vi "Anti-Tip Log.vi"   [LabVIEW 2014]
uses:
  <vilib>/Rock Robotics/Network Tables/SD Read Boolean.vi
  Begin/Global Variables.vi
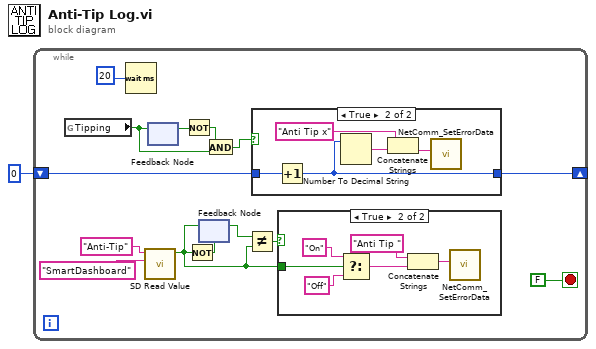
[diagram p0: block diagram]
diagram:
  n1 = while {
    shift-right: [w9] -> _
    shift-left: i16 0 ("width (-)") -> [w10]
    stop <- FALSE stop-if-true
    n2 = global read "Global Variables.vi" "Tipping"() -> (w13:bool)
    n3 = Wait (ms)(milliseconds to wait=u32 20) -> ()  [unwired: 1 out]
    n4 = call-poly <vilib>:"SD Read Value.vi"("Table Prefix"="SmartDashboard", "Name"="Anti-Tip") -> ("Boolean"=w2:bool)  [unwired: 7 in, 2 out]
    n5 = feedback-in #1(w13) -> ()
    n6 = feedback #1() -> (w15:bool)  [unwired: 1 in]
    n7 = Not(x=w15) -> (.not. x?=w14:bool)
    n8 = Not(x=w2) -> (.not. x?=w3:bool)
    n9 = feedback #2(w3) -> (w5:bool)
    n10 = feedback-in #2(w2) -> ()
    n11 = And(x=w14, y=w13) -> (x .and. y?=w12:bool)
    n12 = Not Equal?(x=w5, y=w2) -> (x != y?=w4:bool)
    n13 = case shown="True" w12 {
      tunnel: w10 -> [w22 w24]
      tunnel: [w22 w23] -> w9
      frame False {
      }
      frame True {
        n14 = Increment(x=w24) -> (x+1=w23:i16)
        n15 = Number To Decimal String(number=w23) -> (decimal integer string=w25:string)  [unwired: 1 in]
        n16 = Concatenate Strings("Anti Tip x" ("Error Data"), w25) -> (w26:string)
        n17 = call <vilib>:"NetComm_SetErrorData.vi"("Error Data"=w26) -> ()  [unwired: 3 in, 8 out]
      }
    }
    n18 = case shown="True" w4 {
      tunnel: w2 -> [_ w20]
      frame False {
      }
      frame True {
        n19 = Select(t="On", s=w20, f="Off") -> (s? t:f=w19:string)
        n20 = Concatenate Strings("Anti Tip " ("string"), w19) -> (w21:string)
        n21 = call <vilib>:"NetComm_SetErrorData.vi"("Error Data"=w21) -> ()  [unwired: 3 in, 8 out]
      }
    }
  }
